vi "Populate Recorder List.vi"(4 "Seconds between samples":dbl=1.0 format="%_4f", 6 "Channels to scan (empty - don't use scanner option)":i32[](array[numeric]), 8 "error in (no error)":errorcluster, 11 "VISA Resourse Names":refnum<visa-resource-name>[](array[refnum])) -> (0 "error out":errorcluster, 2 "Names":string[](array[string]), 3 "Instrument List":refnum<class "Instrument Actor.lvclass">[](array[class]))   [LabVIEW 2016]
uses:
  Measure_core/Instrument Actor/Instrument Actor.lvclass
  NHMFL_Core/Libraries/Instruments/Device/Device type.ctl
  Temperature Controller/Temperature Controller.lvclass
  C:/github/Measure_core/Instrument Actor/Instrument Actor.lvclass
  NHMFL_Core/Libraries/Instruments/Cryo-con/Cryo-Con Driver/Cryo-Con Driver.lvclass
  C:/github/NHMFL_Core/Libraries/Instruments/VISA Instrument/VISA Instrument.lvclass
  C:/github/NHMFL_Core/Libraries/Instruments/Instrument Driver/Instrument Driver.lvclass
  C:/github/NHMFL_Core/Libraries/Instruments/Temperature Controller Driver/Temperature Controller Driver.lvclass
  NHMFL_Core/Libraries/Instruments/VISA Instrument/VISA Instrument.lvclass/VISA Instrument.ctl
  NHMFL_Core/Libraries/Instruments/Instrument Driver/Instrument Driver.lvclass/Instrument Driver.ctl
  NHMFL_Core/Libraries/Instruments/Neocera/Neocera Driver/Neocera Driver.lvclass
  NHMFL_Core/Libraries/Instruments/LakeShore/LakeShore T Controller Driver/LakeShore T Controller Driver.lvclass
  Channel Scanner/Channel Scanner.lvclass
  NHMFL_Core/Libraries/Instruments/LR-700/LR-700 Driver/LR-700 Driver.lvclass
  Measure_core/Instrument Actor/Instrument Actor.lvclass/Instrument Actor.ctl
  NHMFL_Core/Libraries/Instruments/Oxford/Oxford PS Driver/Oxford PS Driver.lvclass
  NHMFL_Core/Libraries/Instruments/AH/Andeen-Hagerling Driver/Andeen-Hagerling Driver.lvclass
  NHMFL_Core/Libraries/Instruments/Keithley/Keithley Driver/Keithley Driver.lvclass
  NHMFL_Core/Libraries/Instruments/LakeShore/LakeShore 370 Driver/LakeShore 370 Driver.lvclass
  NHMFL_Core/Libraries/Instruments/SRS/SRS Lockin Driver/SRS Lockin Driver.lvclass
  NHMFL_Core/Libraries/Instruments/VISA Instrument/Write VISA resource.vi
  NHMFL_Core/Libraries/Instruments/Instrument Driver/Write Recorder name.vi
  Measure_core/Instrument Actor/Write Instrument driver.vi
  Temperature Controller/Write T ctl driver.vi
panel:
  in  "Instrument":T1=enum."LkShr 340 chA&B"
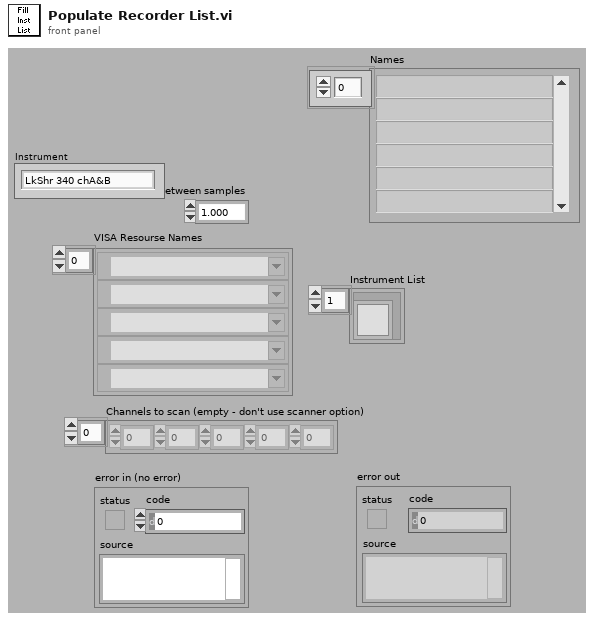
[diagram p1: front panel]
types:
  T1 = typedef "Device type.ctl" = enum16{"NONE", "Neocera 21", "LakeShore 335", "LakeShore 340", "LkShr 340 chA&B", "LakeShore 370", "SRS 850", "SRS 830", "LR 700", "EG&G 5302", "EG&G 7260", "EG&G 7280", "AH 2500", "Keithley meter", "Keithley electrometer", "Keithley 182", "HP 5385", "HP 53181", "HP 53132", "ITC503", "IPS120", "Oxford Mercury IPS", "Oxford PS", "Test", "DC Facility Magnet", "Cryomagnetics PS", "Keithley 2400", "Keithley current source", "Cryo-Con 22C", "HP87NN", "HP4395A"}
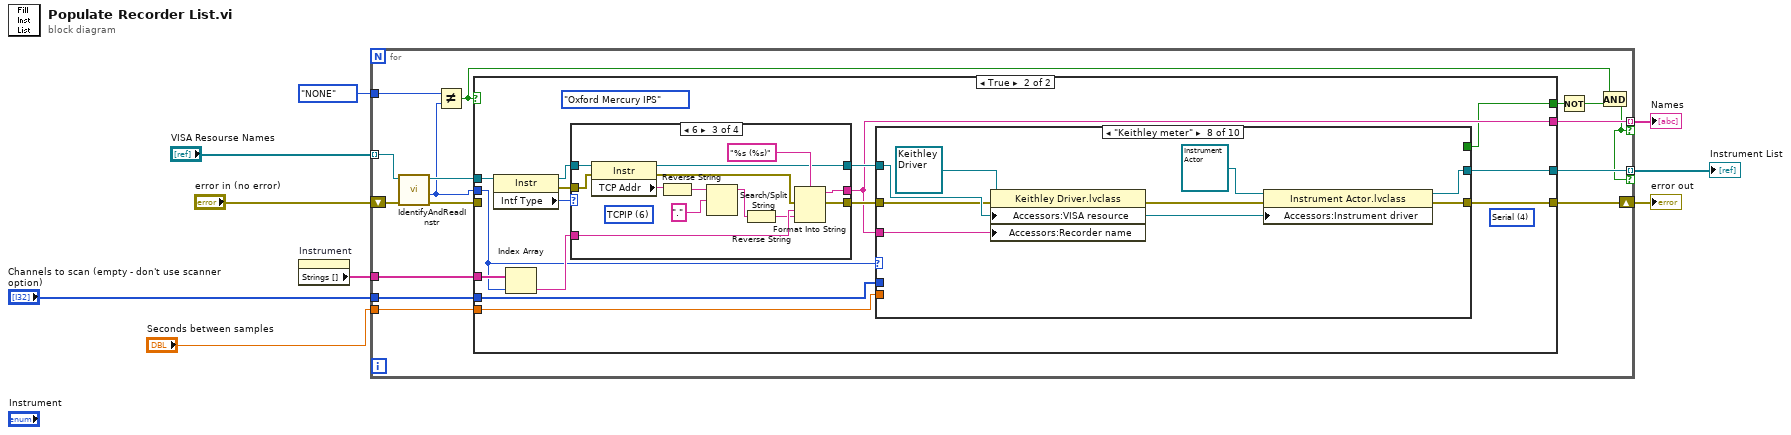
[diagram p0: block diagram]
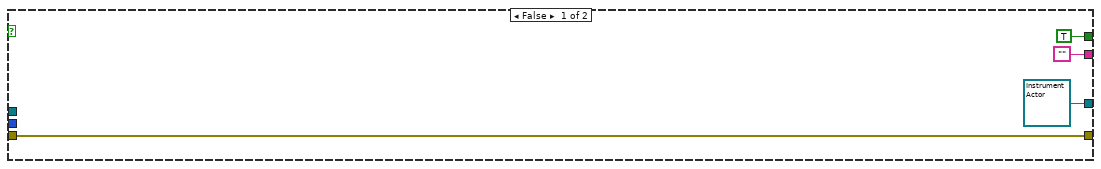
[diagram p2: hidden frame]
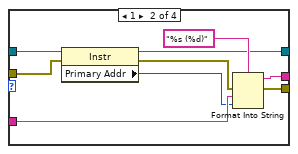
[diagram p4: hidden frame]
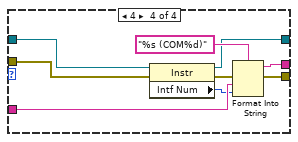
[diagram p5: hidden frame]
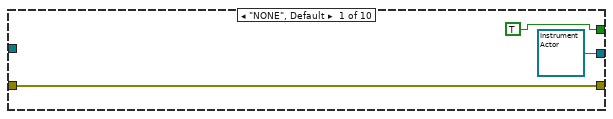
[diagram p6: hidden frame]
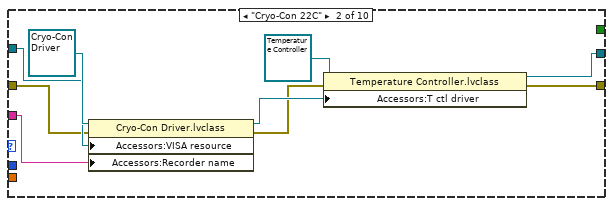
[diagram p7: hidden frame]
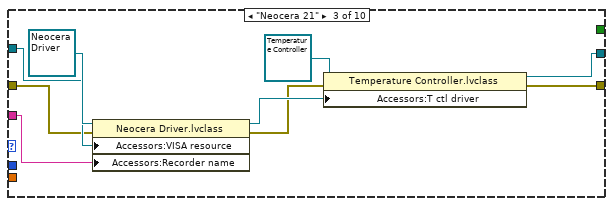
[diagram p8: hidden frame]
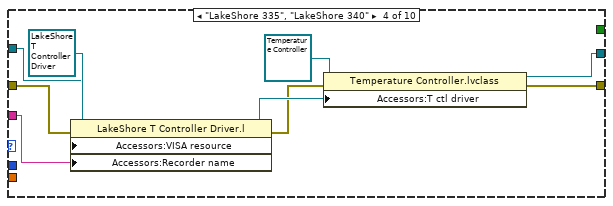
[diagram p9: hidden frame]
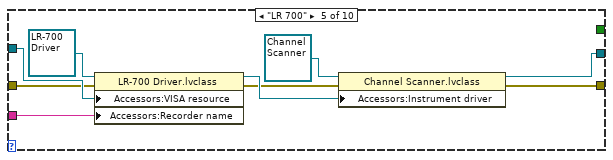
[diagram p10: hidden frame]
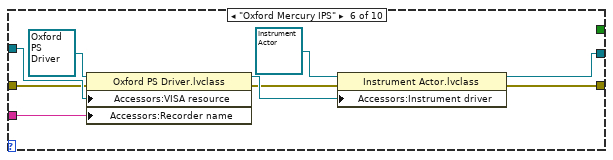
[diagram p11: hidden frame]
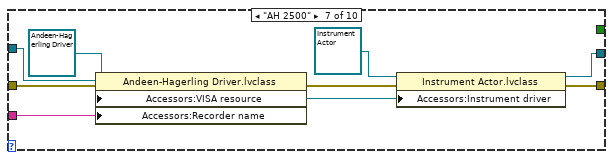
[diagram p12: hidden frame]
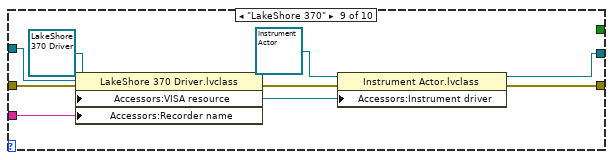
[diagram p13: hidden frame]
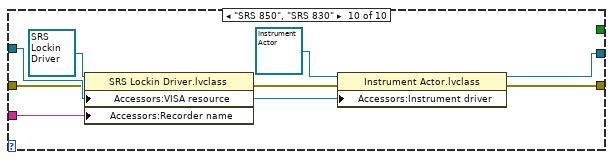
[diagram p14: hidden frame]
diagram:
  n1 = property on="Instrument" class="Enum (strict)"() -> ("Strings []"=w4:string[])  [unwired: 2 in, 2 out]
  n2 = for {
    tunnel: "VISA Resourse Names" -> [w23] mode=indexing
    shift-right: [w19] -> w7
    shift-left: "error in (no error)" -> [w25]
    tunnel: "Channels to scan (empty - don't use scanner option)" -> [w22]
    tunnel: "Seconds between samples" -> [w21]
    tunnel: w4 -> [w16]
    tunnel: Device_type."NONE" ("Instrument") -> [w18]
    tunnel: [w15] -> w2 mode=indexing if=w12
    tunnel: [w14] -> w1 mode=indexing if=w12
    n3 = call "IdentifyAndReadInstr.vi"("error in (no error)"=w25, "VISA Resource Name"=w23) -> ("error out"=w24:errorcluster, "Instrument"=w17:T1, "VISA Resource Name Out"=w20:refnum<visa-resource-name>)  [unwired: 6 in, 1 out]
    n4 = Not Equal?(x=w18, y=w17) -> (x != y?=w13:bool)
    n5 = case shown="True" w13 {
      tunnel: w24 -> [w29 _]
      tunnel: w22 -> [_ w44]
      tunnel: w21 -> [_ w43]
      tunnel: w20 -> [_ w38]
      tunnel: w17 -> [_ w40]
      tunnel: [refnum<class "Instrument Actor.lvclass"> refnum ("Instrument Recorder.lvclass") w35] -> w15
      tunnel: [w29 w32] -> w19
      tunnel: w16 -> [_ w42]
      tunnel: ["" w31] -> w14
      tunnel: [TRUE w30] -> w11
      frame False {
      }
      frame True {
        (unwired) Device_type."Oxford Mercury IPS" ("Instrument")
        (unwired) u16 4 items=["GPIB"=1, "VXI"=2, "GPIB-VXI"=3, "Serial"=4, "PXI"=5, "TCPIP"=6, "USB"=7, "FireWire"=9] ("Interface Information:Interface Type")
        n6 = property class="Instr"(reference=w38) -> (reference out=w39:refnum<visa-resource-name>, error out=w37:errorcluster, "Intf Type"=w36:u16)  [unwired: 1 in]
        n7 = Index Array(array=w42, index=w40) -> (element=w41:string)
        n8 = case shown="6" w36 {
          tunnel: w41 -> [w45 w54 w67 w76]
          tunnel: [w46 w52 w66 w70] -> w33
          tunnel: [w45 w51 w65 w74] -> w31
          tunnel: [w47 w50 w64 w73] -> w34
          tunnel: w39 -> [w46 w49 w63 w72]
          tunnel: w37 -> [w47 w48 w62 w71]
          frame 0, Default {
          }
          frame 1 {
            n9 = property class="Instr"(reference=w49, error in=w48) -> (reference out=w52:refnum<visa-resource-name>, error out=w56:errorcluster, "Primary Addr"=w53:u16)
            n10 = Format Into String(format string="%s (%d)", error in=w56, w54, w53) -> (resulting string=w51:string, error out=w50:errorcluster)  [unwired: 1 in]
          }
          frame 6 {
            (unwired) u16 6 items=["GPIB"=1, "VXI"=2, "GPIB-VXI"=3, "Serial"=4, "PXI"=5, "TCPIP"=6, "USB"=7, "FireWire"=9] ("Interface Information:Interface Type")
            n11 = property class="Instr"(reference=w63, error in=w62) -> (reference out=w66:refnum<visa-resource-name>, error out=w69:errorcluster, "TCP Addr"=w61:string)
            n12 = Reverse String(1:w61) -> (0:w59:string)
            n13 = Search/Split String(string=w59, search string/char (-)="." ("regular expression")) -> (substring before match=w58:string)  [unwired: 1 in, 2 out]
            n14 = Reverse String(1:w58) -> (0:w60:string)
            n15 = Format Into String(format string="%s (%s)", error in=w69, w67, w60) -> (resulting string=w65:string, error out=w64:errorcluster)  [unwired: 1 in]
          }
          frame 4 {
            n16 = property class="Instr"(reference=w72, error in=w71) -> (reference out=w70:refnum<visa-resource-name>, error out=w78:errorcluster, "Intf Num"=w75:u16)
            n17 = Format Into String(format string="%s (COM%d)", error in=w78, w76, w75) -> (resulting string=w74:string, error out=w73:errorcluster)  [unwired: 1 in]
          }
        }
        n18 = case shown="\"Keithley meter\"" w40 {
          tunnel: w34 -> [w81 w84 w93 w102 w111 w121 w130 w139 w148 w157]
          tunnel: [w81 w83 w92 w101 w110 w120 w129 w138 w147 w156] -> w32
          tunnel: [refnum<class "Instrument Actor.lvclass"> refnum ("Instrument Recorder.lvclass") w89 w98 w107 w113 w123 w132 w141 w150 w159] -> w35
          tunnel: w44 -> [_ _ _ _ _ _ _ _ _ _]
          tunnel: w43 -> [_ _ _ _ _ _ _ _ _ _]
          tunnel: w33 -> [_ w86 w95 w104 w115 w124 w133 w142 w151 w160]
          tunnel: w31 -> [_ w82 w91 w100 w109 w119 w128 w137 w146 w155]
          tunnel: [TRUE _ _ _ _ _ _ _ _ _] -> w30
          frame "NONE", Default {
          }
          frame "Cryo-Con 22C" {
            n19 = property class="Cryo-Con Driver.lvclass"(reference=refnum<class "Cryo-Con Driver.lvclass"> refnum ("Cryo-Con Driver.lvclass"), error in=w84, "Accessors:VISA resource"=w86, "Accessors:Recorder name"=w82) -> (reference out=w87:refnum<class "Cryo-Con Driver.lvclass">, error out=w85:errorcluster)
            n20 = property class="Temperature Controller.lvclass"(reference=refnum<class "Temperature Controller.lvclass"> refnum ("Temperature Controller.lvclass"), error in=w85, "Accessors:T ctl driver"=w87) -> (reference out=w89:refnum<class "Temperature Controller.lvclass">, error out=w83:errorcluster)
          }
          frame "Neocera 21" {
            n21 = property class="Neocera Driver.lvclass"(reference=refnum<class "Neocera Driver.lvclass"> refnum ("Neocera Driver.lvclass"), error in=w93, "Accessors:VISA resource"=w95, "Accessors:Recorder name"=w91) -> (reference out=w96:refnum<class "Neocera Driver.lvclass">, error out=w94:errorcluster)
            n22 = property class="Temperature Controller.lvclass"(reference=refnum<class "Temperature Controller.lvclass"> refnum ("Temperature Controller.lvclass"), error in=w94, "Accessors:T ctl driver"=w96) -> (reference out=w98:refnum<class "Temperature Controller.lvclass">, error out=w92:errorcluster)
          }
          frame "LakeShore 335", "LakeShore 340" {
            n23 = property class="LakeShore T Controller Driver.l"(reference=refnum<class "LakeShore T Controller Driver.lvclass"> refnum ("LakeShore T Controller Driver.lvclass"), error in=w102, "Accessors:VISA resource"=w104, "Accessors:Recorder name"=w100) -> (reference out=w105:refnum<class "LakeShore T Controller Driver.lvclass">, error out=w103:errorcluster)
            n24 = property class="Temperature Controller.lvclass"(reference=refnum<class "Temperature Controller.lvclass"> refnum ("Temperature Controller.lvclass"), error in=w103, "Accessors:T ctl driver"=w105) -> (reference out=w107:refnum<class "Temperature Controller.lvclass">, error out=w101:errorcluster)
          }
          frame "LR 700" {
            n25 = property class="LR-700 Driver.lvclass"(reference=refnum<class "LR-700 Driver.lvclass"> refnum ("LR-700 Driver.lvclass"), error in=w111, "Accessors:VISA resource"=w115, "Accessors:Recorder name"=w109) -> (reference out=w116:refnum<class "LR-700 Driver.lvclass">, error out=w112:errorcluster)
            n26 = property class="Channel Scanner.lvclass"(reference=refnum<class "Channel Scanner.lvclass"> refnum ("Channel Scanner.lvclass"), error in=w112, "Accessors:Instrument driver"=w116) -> (reference out=w113:refnum<class "Channel Scanner.lvclass">, error out=w110:errorcluster)
          }
          frame "Oxford Mercury IPS" {
            n27 = property class="Oxford PS Driver.lvclass"(reference=refnum<class "Oxford PS Driver.lvclass"> refnum ("Oxford PS Driver.lvclass"), error in=w121, "Accessors:VISA resource"=w124, "Accessors:Recorder name"=w119) -> (reference out=w125:refnum<class "Oxford PS Driver.lvclass">, error out=w122:errorcluster)
            n28 = property class="Instrument Actor.lvclass"(reference=refnum<class "Instrument Actor.lvclass"> refnum ("Instrument Recorder.lvclass"), error in=w122, "Accessors:Instrument driver"=w125) -> (reference out=w123:refnum<class "Instrument Actor.lvclass">, error out=w120:errorcluster)
          }
          frame "AH 2500" {
            n29 = property class="Andeen-Hagerling Driver.lvclass"(reference=refnum<class "Andeen-Hagerling Driver.lvclass"> refnum ("Andeen-Hagerling Driver.lvclass"), error in=w130, "Accessors:VISA resource"=w133, "Accessors:Recorder name"=w128) -> (reference out=w134:refnum<class "Andeen-Hagerling Driver.lvclass">, error out=w131:errorcluster)
            n30 = property class="Instrument Actor.lvclass"(reference=refnum<class "Instrument Actor.lvclass"> refnum ("Instrument Recorder.lvclass"), error in=w131, "Accessors:Instrument driver"=w134) -> (reference out=w132:refnum<class "Instrument Actor.lvclass">, error out=w129:errorcluster)
          }
          frame "Keithley meter" {
            n31 = property class="Keithley Driver.lvclass"(reference=refnum<class "Keithley Driver.lvclass"> refnum ("Keithley Driver.lvclass"), error in=w139, "Accessors:VISA resource"=w142, "Accessors:Recorder name"=w137) -> (reference out=w143:refnum<class "Keithley Driver.lvclass">, error out=w140:errorcluster)
            n32 = property class="Instrument Actor.lvclass"(reference=refnum<class "Instrument Actor.lvclass"> refnum ("Instrument Recorder.lvclass"), error in=w140, "Accessors:Instrument driver"=w143) -> (reference out=w141:refnum<class "Instrument Actor.lvclass">, error out=w138:errorcluster)
          }
          frame "LakeShore 370" {
            n33 = property class="LakeShore 370 Driver.lvclass"(reference=refnum<class "LakeShore 370 Driver.lvclass"> refnum ("LakeShore 370 Driver.lvclass"), error in=w148, "Accessors:VISA resource"=w151, "Accessors:Recorder name"=w146) -> (reference out=w152:refnum<class "LakeShore 370 Driver.lvclass">, error out=w149:errorcluster)
            n34 = property class="Instrument Actor.lvclass"(reference=refnum<class "Instrument Actor.lvclass"> refnum ("Instrument Recorder.lvclass"), error in=w149, "Accessors:Instrument driver"=w152) -> (reference out=w150:refnum<class "Instrument Actor.lvclass">, error out=w147:errorcluster)
          }
          frame "SRS 850", "SRS 830" {
            n35 = property class="SRS Lockin Driver.lvclass"(reference=refnum<class "SRS Lockin Driver.lvclass"> refnum ("SRS Lockin Driver.lvclass"), error in=w157, "Accessors:VISA resource"=w160, "Accessors:Recorder name"=w155) -> (reference out=w161:refnum<class "SRS Lockin Driver.lvclass">, error out=w158:errorcluster)
            n36 = property class="Instrument Actor.lvclass"(reference=refnum<class "Instrument Actor.lvclass"> refnum ("Instrument Recorder.lvclass"), error in=w158, "Accessors:Instrument driver"=w161) -> (reference out=w159:refnum<class "Instrument Actor.lvclass">, error out=w156:errorcluster)
          }
        }
      }
    }
    n37 = Not(x=w11) -> (.not. x?=w10:bool)
    n38 = And(x=w13, y=w10) -> (x .and. y?=w12:bool)
  }
  "error out" <- w7
  "Instrument List" <- w2
  "Names" <- w1
